vi "Cumulative.vi"() -> ()   [LabVIEW 2017]
uses:
  <vilib>/vision/NI_Vision_Development_Module.lvlib
panel:
  out "Image":T1(plugin-control)
  out "Minimal Value":sgl
  out "Maximal Value":sgl
  out "Cumulative Histogram":dbl[](graph)
  out "Histogram":T2(graph)
  out "90%":dbl
  out "10%":dbl
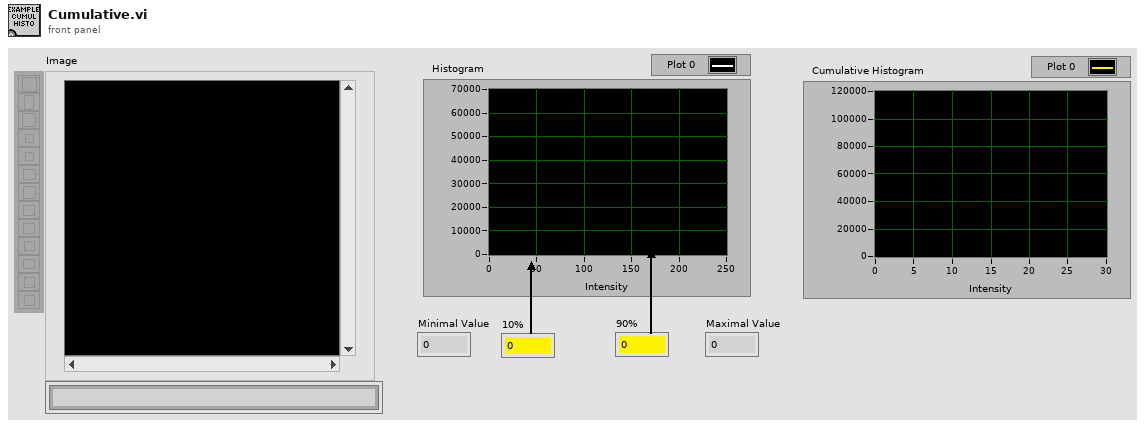
[diagram p1: front panel]
types:
  T1 = typedef "IMAQ Image.ctl" = refnum<image>
  T2 = cluster{"Starting Value":sgl, "Incremental Value":sgl, "Histogram":u32[]}
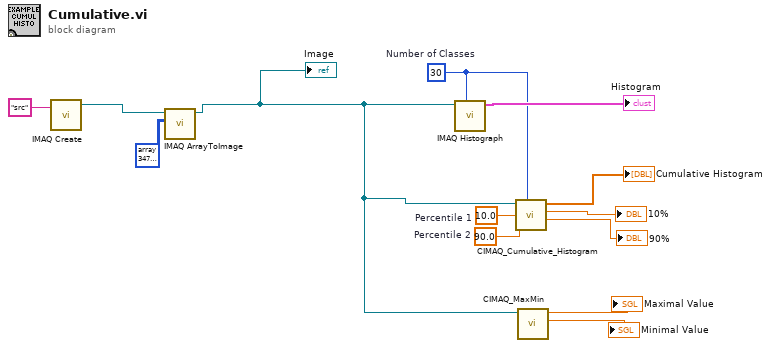
[diagram p0: block diagram]
diagram:
  w6 = 30  # Number of Classes
  w11 = sgl 90.0  # Percentile 2
  w12 = sgl 10.0  # Percentile 1
  n1 = call "IMAQ Create"("Image Name"="src") -> ("New Image"=w3:T1)  [unwired: 4 in, 1 out]
  n2 = call "IMAQ ArrayToImage"("Image Pixels (U8)"=u8[][] array347x337[116939 elements], "Image"=w3) -> ("Image Out"=w2:T1)  [unwired: 8 in, 1 out]
  "Image" <- w2
  n3 = call "IMAQ Histograph"("Number of Classes"=w6, "Image"=w2) -> ("Histogram Graph"=→"Histogram":T2)  [unwired: 6 in, 3 out]
  n4 = call "CIMAQ_Cumulative_Histogram.vi"("Img"=w2, "Percentile 1"=w12, "Percentile 2"=w11, "Number of Classes"=w6) -> ("Cumulative Histogram"=→"Cumulative Histogram":dbl[], "Percentile 1"=→"10%":sgl, "Percentile 2"=→"90%":sgl)  [unwired: 3 in, 1 out]
  n5 = call <userlib>:"CIMAQ_MaxMin.vi"("Img In"=w2) -> ("Minimal Value"=→"Minimal Value":sgl, "Maximal Value"=→"Maximal Value":sgl)  [unwired: 8 in, 1 out]
